vi "_free.vi"(9 "error in (no error)":errorcluster, 10 "MDPtr DVR":refnum<data-value>) -> (2 "error out":errorcluster)   [LabVIEW 2017, in "MDPtr.lvlib"]
uses:
  MDPtr.lvlib
  MDPtr TypeDef/MDPtr DataFrame-Memory.ctl
  MDPtr TypeDef/MDPtr DataFrame-Common.ctl
  <vilib>/Utility/Data Type/Type Definitions/Data Type.ctl
  _MDPtr Build Error Cluster.vi
  <vilib>/Utility/Data Type/NI_Data Type.lvlib
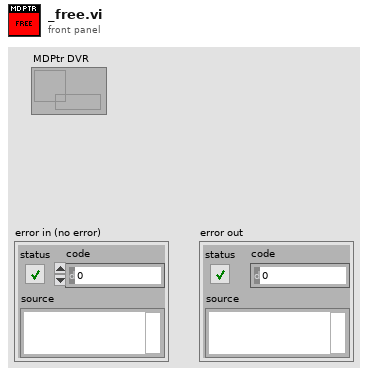
[diagram p1: front panel]
types:
  T1 = typedef "MDPtr.lvlib/MDPtr DataFrame-Memory.ctl" = cluster{"Common":T2, "DVR":refnum<data-value>}
  T2 = typedef "MDPtr.lvlib/MDPtr DataFrame-Common.ctl" = cluster{"Data Type":T3, "Copy Count":i32, "String Attribute":string, "Cache Length":i32, "Data Length":i32}
  T3 = typedef "NI_Data Type.lvlib/Data Type.ctl" = enum8{"Invalid Type", "Void", "I8", "I16", "I32", "I64", "U8", "U16", "U32", "U64", "Single Float", "Double Float", "Extended Float", "Single Complex", "Double Complex", "Extended Complex", "Enum U8", "Enum U16", "Enum U32", "Enum U64", "Single Float With Unit", "Double Float With Unit", "Extended Float With Unit", "Single Complex with Unit", "Double Complex with Unit", "Extended Complex with Unit", "Boolean", "String", "Path", "Picture", "Tag", "Array", "Cluster", "Variant", "LV Variant", "Waveform", "Timestamp", "Digital Waveform", "Digital Data", "ExpressData", "Refnum", "External Data", "VI", "Poly VI", "LabVIEW Class Instance", "Fixed Point"}
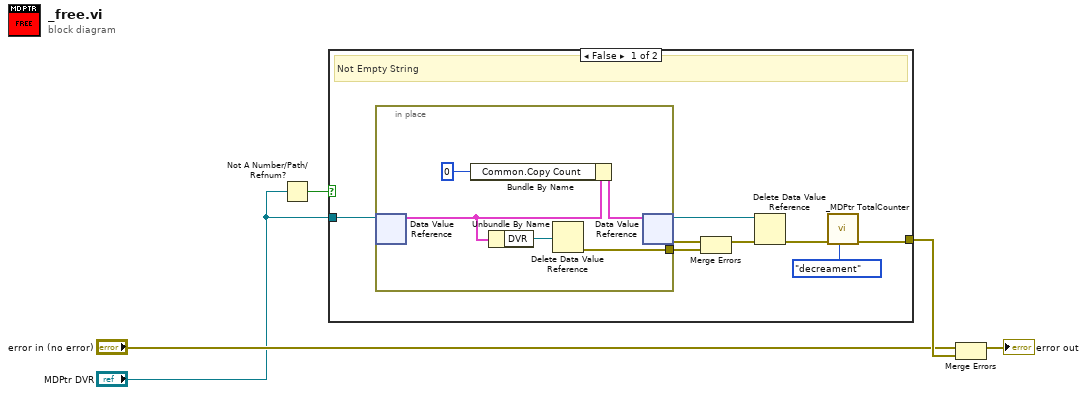
[diagram p0: block diagram]
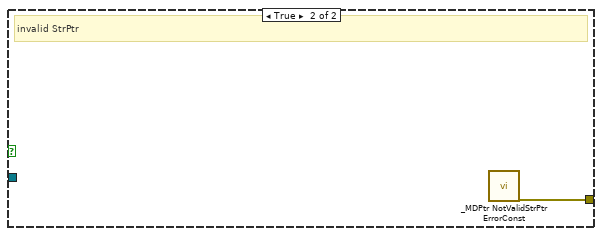
[diagram p2: hidden frame]
diagram:
  n1 = Not A Number/Path/Refnum?(number/path/refnum="MDPtr DVR") -> (NaN/Path/Refnum?=w1:bool)
  n2 = case shown="False" w1 {
    tunnel: [w7 w19] -> w5
    tunnel: "MDPtr DVR" -> [w12 _]
    frame False {
      # "Not Empty String"
      n3 = in-place {
        in-place-border: [w14] -> w8
        n4 = in-place-dvr #1(w12) -> (w18:T1)  [unwired: 1 out]
        n5 = Bundle By Name(cluster=w18, "Common.Copy Count"=0) -> (w17:T1)
        n6 = Unbundle By Name(w18) -> ("DVR"=w15:refnum<data-value>)
        n7 = Delete Data Value Reference(data value reference=w15) -> (error out=w14:errorcluster)  [unwired: 1 in, 1 out]
        n8 = in-place-dvr #1(w17) -> (w10:refnum<data-value>, w13:errorcluster)
      }
      n9 = Merge Errors(w13, w8) -> (w9:errorcluster)
      n10 = Delete Data Value Reference(data value reference=w10, error in=w9) -> (error out=w11:errorcluster)  [unwired: 1 out]
      n11 = call "_MDPtr TotalCounter.vi"("Oper(Get)"=enum16{"GET", "Increament", "decreament"}."decreament", "error in (no error)"=w11) -> ("error out"=w7:errorcluster)  [unwired: 8 in, 1 out]
    }
    frame True {
      # "invalid StrPtr"
      n12 = call "_MDPtr NotValidStrPtr ErrorConst.vi"() -> ("error out"=w19:errorcluster)  [unwired: 19 in]
    }
  }
  n13 = Merge Errors("error in (no error)", w5) -> (→"error out":errorcluster)
